vi "实验4_4.vi"() -> ()   [LabVIEW 2018]
panel:
  out "Intensity Graph":dbl[][](graph)
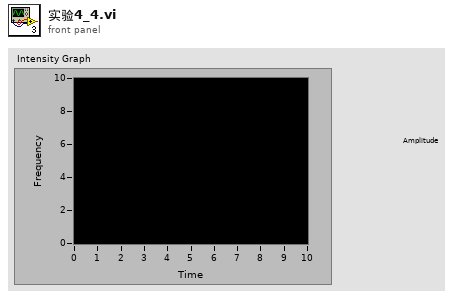
[diagram p1: front panel]
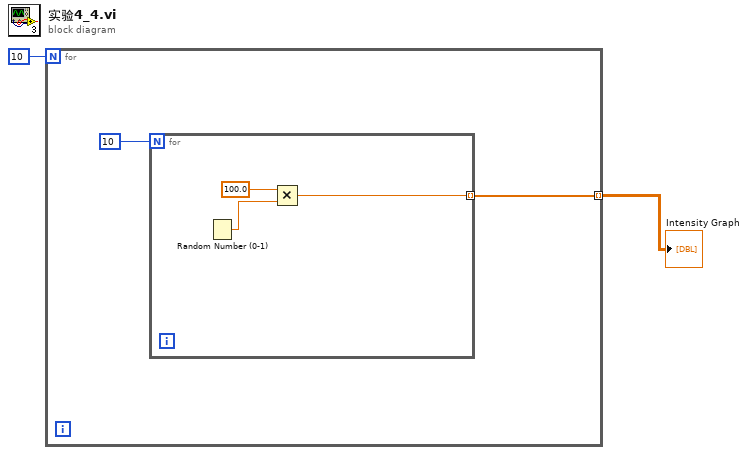
[diagram p0: block diagram]
diagram:
  n1 = for {
    N: 10 -> [_]
    tunnel: [w3] -> w1 mode=indexing
    n2 = for {
      N: 10 -> [_]
      tunnel: [w5] -> w3 mode=indexing
      n3 = Random Number (0-1)() -> (number: 0 to 1=w6:dbl)
      n4 = Multiply(x=100.0, y=w6) -> (x*y=w5:dbl)
    }
  }
  "Intensity Graph" <- w1
